vi "manual test UI.vi"(8 "error in (no error)":errorcluster caption="Fehler (Eingang, kein Fehler)", 11 "Stoeraussendung Eingang":refnum<class "Stoeraussendung.lvclass"> caption="DNL_LabVIEW Object in") -> (0 "error out":errorcluster caption="Fehler (Ausgang)", 1 "parameters":string[][](table), 2 "Parameters":u32[](array[numeric]), 3 "Stoeraussendung Ausgang":refnum<class "Stoeraussendung.lvclass"> caption="DNL_LabVIEW Object out", 5 "abbrechen":bool)   [LabVIEW 2013, in "Stoeraussendung.lvclass"]
uses:
  Stoeraussendung.lvclass
panel:
  in  "Abbrechen":bool
  in  "OK Button":bool
  in  "Radio Buttons":enum32{"DPX", "AVG", "QPK"}(radio)
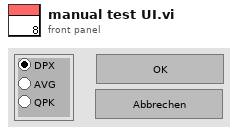
[diagram p1: front panel]
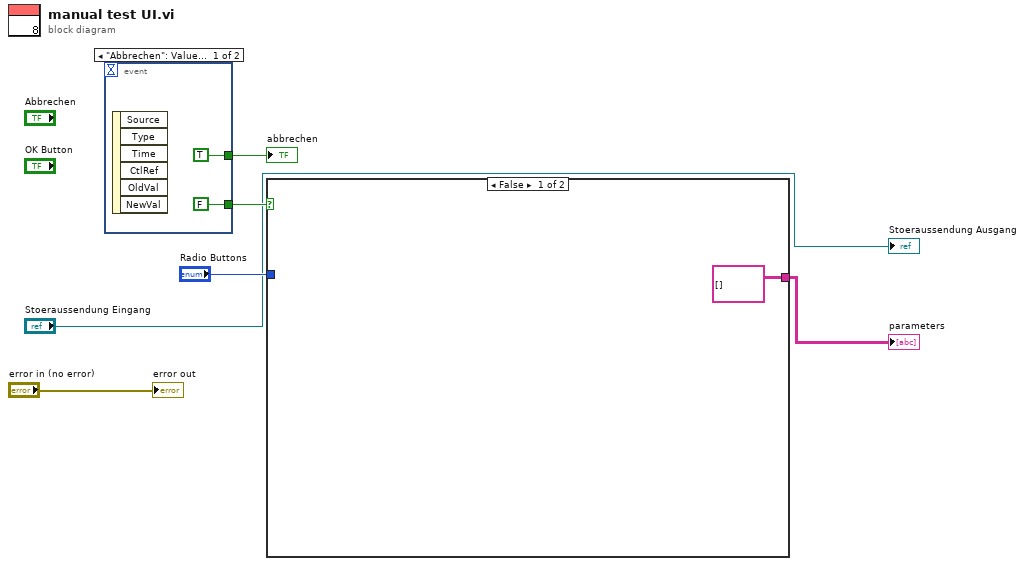
[diagram p0: block diagram]
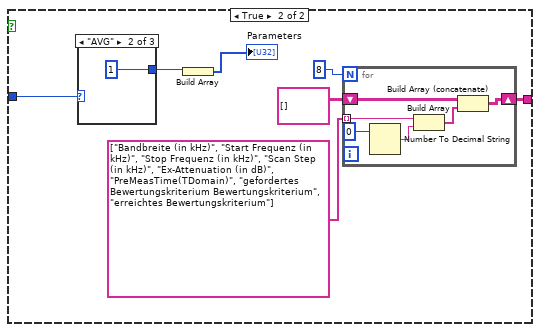
[diagram p2: hidden frame]
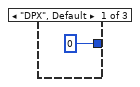
[diagram p3: hidden frame]
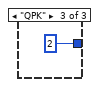
[diagram p4: hidden frame]
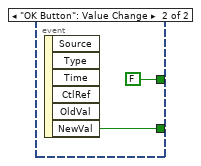
[diagram p5: hidden frame]
diagram:
  n1 = event shown="[0] \"Abbrechen\": Value Change" {
    selector: _ -> [_ _]
    dyn-events: _ -> [_ _]
    timeout: _ -> [_ _]
    tunnel: [TRUE ("abbrechen") FALSE ("abbrechen")] -> w5
    tunnel: [FALSE ("NewVal") w9] -> w4
    event "Abbrechen": Value Change {
      n2 = event-data() -> ()  [unwired: 1 in, 6 out]
    }
    event "OK Button": Value Change {
      n3 = event-data() -> ("NewVal"=w9:bool)  [unwired: 1 in, 5 out]
    }
  }
  "abbrechen" <- w5
  n4 = case shown="False" w4 {
    tunnel: "Radio Buttons" -> [_ w18]
    tunnel: [string[][] [] w13] -> w3
    frame False {
    }
    frame True {
      n5 = case shown="\"AVG\"" w18 {
        tunnel: [u32 0 u32 1 u32 2] -> w15
        frame "DPX", Default {
        }
        frame "AVG" {
        }
        frame "QPK" {
        }
      }
      n6 = Build Array(w15) -> (→"Parameters":u32[])
      n7 = for {
        N: 8 -> [_]
        tunnel: string[] ["Bandbreite (in kHz)", "Start Frequenz (in kHz)", "Stop Frequenz (in kHz)", "Scan Step (in kHz)", "Ex-Attenuation (in dB)", "PreMeasTime(TDomain)", "gefordertes Bewertungskriterium Bewertungskriterium", "erreichtes Bewertungskriterium"] -> [w24] mode=indexing
        shift-right: [w20] -> w13
        shift-left: string[][] [] -> [w22]
        n8 = Number To Decimal String(number=0) -> (decimal integer string=w23:string)  [unwired: 1 in]
        n9 = Build Array(w24, w23) -> (w21:string[])
        n10 = Build Array (concatenate)(w22, w21) -> (w20:string[][])
      }
    }
  }
  "parameters" <- w3
  "error out" <- "error in (no error)"
  "Stoeraussendung Ausgang" <- "Stoeraussendung Eingang"
